vi "Special Read.vi"(8 "error in (no error)":errorcluster, 11 "VISA resource name":refnum<visa-resource-name>) -> (0 "error out":errorcluster, 2 "Output String":string, 3 "VISA resource name out":refnum<visa-resource-name>)   [LabVIEW 2015, in "Ohaus AV Series.lvlib"]
doc: "This VI reads data from the balance's output buffer. It will continue to read until a \\r\\n is recieved. s"
uses:
  Ohaus AV Series.lvlib
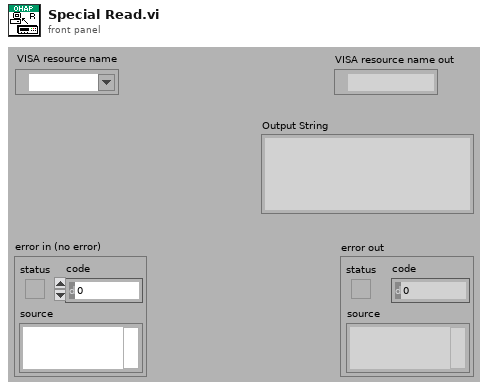
[diagram p1: front panel]
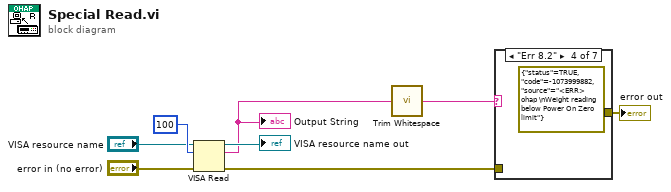
[diagram p0: block diagram]
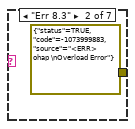
[diagram p3: hidden frame]
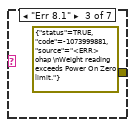
[diagram p4: hidden frame]
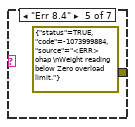
[diagram p5: hidden frame]
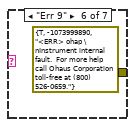
[diagram p6: hidden frame]
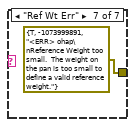
[diagram p7: hidden frame]
diagram:
  n1 = VISA Read(VISA resource name="VISA resource name", byte count=u32 100, error in (no error)="error in (no error)") -> (VISA resource name out=→"VISA resource name out":refnum<visa-resource-name>, read buffer=w3:string, error out=w1:errorcluster)  [unwired: 1 out]
  "Output String" <- w3
  n2 = call <vilib>:"Trim Whitespace.vi"("string"=w3) -> ("trimmed string"=w7:string)  [unwired: 1 in]
  n3 = case shown="\"Err 8.2\"" w7 {
    tunnel: w1 -> [w9 _ _ _ _ _ _]
    tunnel: [w9 errorcluster {"status"=TRUE, "code"=-1073999883, "source"="<ERR> ohap \nOverload Error"} ("error in (no error)") errorcluster {"status"=TRUE, "code"=-1073999881, "source"="<ERR> ohap \nWeight reading exceeds Power On Zero limit."} ("error in (no error)") errorcluster {"status"=TRUE, "code"=-1073999882, "source"="<ERR> ohap \nWeight reading below Power On Zero limit"} ("error in (no error)") errorcluster {"status"=TRUE, "code"=-1073999884, "source"="<ERR> ohap \nWeight reading below Zero overload limit."} ("error in (no error)") errorcluster {"status"=TRUE, "code"=-1073999890, "source"="<ERR> ohap \nInstrument internal fault.  For more help call Ohaus Corporation toll-free at (800) 526-0659."} ("error in (no error)") errorcluster {"status"=TRUE, "code"=-1073999891, "source"="<ERR> ohap\nReference Weight too small.  The weight on the pan is too small to define a valid reference weight."} ("error in (no error)")] -> w6
    frame "False", Default {
    }
    frame "Err 8.3" {
    }
    frame "Err 8.1" {
    }
    frame "Err 8.2" {
    }
    frame "Err 8.4" {
    }
    frame "Err 9" {
    }
    frame "Ref Wt Err" {
    }
  }
  "error out" <- w6
